vi "p8.12.vi"() -> ()   [LabVIEW 2020]
uses:
  <vilib>/vision/NI_Vision_Development_Module.lvlib
panel:
  out "FFT":T1(plugin-control)
  out "Imagen1":T1(plugin-control)
  in  "k2":dbl=1.0
  in  "k1":dbl=1.0
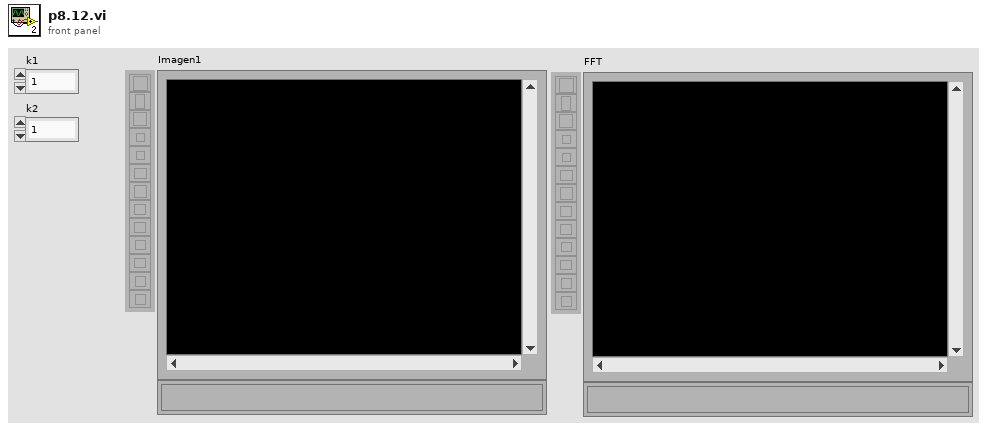
[diagram p1: front panel]
types:
  T1 = typedef "IMAQ Image.ctl" = refnum<image>
  T2 = typedef "Image Type" = u32
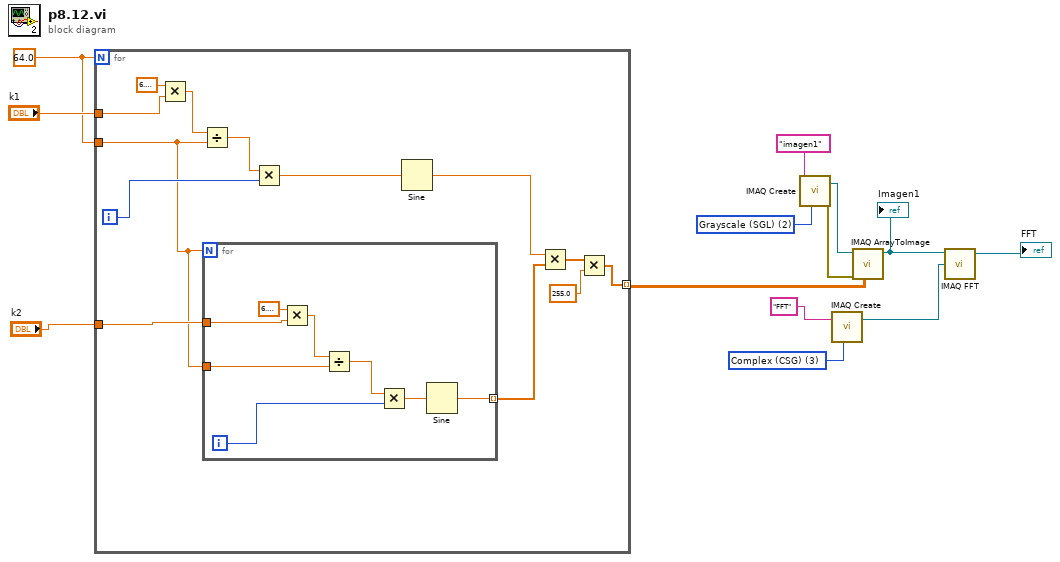
[diagram p0: block diagram]
diagram:
  w3 = T2 3 items=["Grayscale (U8)", "Grayscale (I16)", "Grayscale (SGL)", "Complex (CSG)", "RGB (U32)", "HSL (U32)", "RGB (U64)", "Grayscale (U16)"] ("Image Type")
  w7 = T2 2 items=["Grayscale (U8)", "Grayscale (I16)", "Grayscale (SGL)", "Complex (CSG)", "RGB (U32)", "HSL (U32)", "RGB (U64)", "Grayscale (U16)"] ("Image Type")
  w12 = 64.0 ("y")
  n1 = for {
    N: w12 -> [_]
    tunnel: "k1" -> [w25]
    tunnel: w12 -> [w19]
    tunnel: "k2" -> [w20]
    tunnel: [w14] -> w10 mode=indexing
    i -> [w21]
    n2 = Multiply(x=6.283185307179586, y=w25) -> (x*y=w24:dbl)
    n3 = Divide(x=w24, y=w19) -> (x/y=w23:dbl)
    n4 = for {
      N: w19 -> [_]
      tunnel: [w30] -> w15 mode=indexing
      tunnel: w19 -> [w29]
      tunnel: w20 -> [w28]
      i -> [w27]
      n5 = Multiply(x=6.283185307179586, y=w28) -> (x*y=w33:dbl)
      n6 = Divide(x=w33, y=w29) -> (x/y=w32:dbl)
      n7 = Multiply(x=w32, y=w27) -> (x*y=w31:dbl)
      n8 = Sine(x=w31) -> (sin(x)=w30:dbl)
    }
    n9 = Multiply(x=w23, y=w21) -> (x*y=w22:dbl)
    n10 = Sine(x=w22) -> (sin(x)=w16:dbl)
    n11 = Multiply(x=w16, y=w15) -> (x*y=w18:dbl[])
    n12 = Multiply(x=w18, y=255.0) -> (x*y=w14:dbl[])
  }
  n13 = call "IMAQ Create"("Image Name"="imagen1", "Image Type"=w7) -> ("New Image"=w9:T1, "error out"=w6:errorcluster)  [unwired: 3 in]
  n14 = call "IMAQ Create"("Image Name"="FFT", "Image Type"=w3) -> ("New Image"=w2:T1)  [unwired: 3 in, 1 out]
  n15 = call "IMAQ ArrayToImage"("Image Pixels (Float)"=w10, "error in (no error)"=w6, "Image"=w9) -> ("Image Out"=w5:T1)  [unwired: 7 in, 1 out]
  "Imagen1" <- w5
  n16 = call "IMAQ FFT"("Image Dst"=w2, "Image Src"=w5) -> ("Image Dst Out"=→"FFT":T1)  [unwired: 2 in, 1 out]
